vi "RSZVB Get Source Power Calibration Convergence Factor.vi"(8 "error in (no error)":errorcluster {"code" format="%.0x"}, 11 "VISA session":refnum<visa-resource-name>) -> (0 "error out":errorcluster {"code" format="%.0x"}, 1 "Convergence Factor":dbl format="%^.3e", 3 "dup VISA session":refnum<visa-resource-name>)   [LabVIEW 2011]
doc: "Returns the convergence factor for a source power calibration. \n\nRemote-control command(s):\nSOURce<Ch>:POWer<Pt>:CORRection:COLLect:CFACtor?"
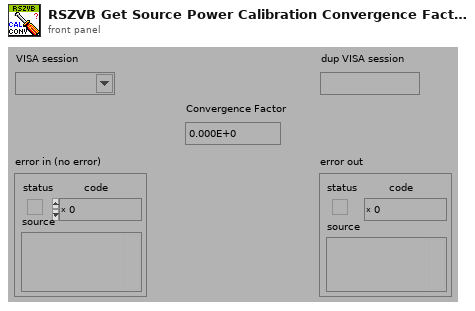
[diagram p1: front panel]
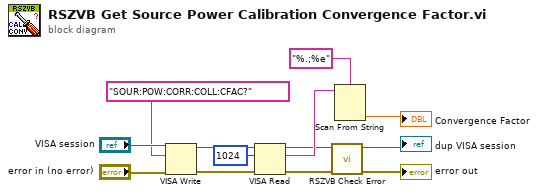
[diagram p0: block diagram]
diagram:
  n1 = VISA Write(VISA resource name="VISA session", write buffer="SOUR:POW:CORR:COLL:CFAC?", error in (no error)="error in (no error)") -> (VISA resource name out=w9:refnum<visa-resource-name>, error out=w10:errorcluster)  [unwired: 1 out]
  n2 = VISA Read(VISA resource name=w9, byte count=u32 1024, error in (no error)=w10) -> (VISA resource name out=w4:refnum<visa-resource-name>, read buffer=w6:string, error out=w5:errorcluster)  [unwired: 1 out]
  n3 = call "RSZVB Check Error.vi"("error in (no error)"=w5, "VISA session"=w4) -> ("error out"=→"error out":errorcluster, "dup VISA session"=→"dup VISA session":refnum<visa-resource-name>)  [unwired: 8 in]
  n4 = Scan From String(format string="%.;%e", input string=w6) -> (output 1=→"Convergence Factor":dbl)  [unwired: 3 in, 3 out]
